vi "CreateNewProj.vi"() -> ()   [LabVIEW 2026]
panel:
  out "error out":errorcluster
  in  "error in (no error)":errorcluster
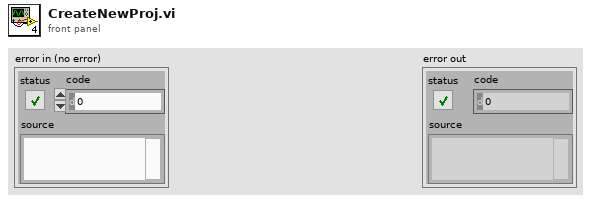
[diagram p1: front panel]
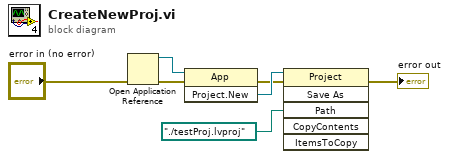
[diagram p0: block diagram]
diagram:
  n1 = Open Application Reference(8:"error in (no error)") -> (0:w3:errorcluster, 3:w7:refnum<vi>)  [unwired: 3 in]
  n2 = invoke class="App" method="Project.New"(reference=w7, error in=w3) -> (error out=w2:errorcluster, "Project:New"=w6:refnum<vi>)  [unwired: 1 in, 1 out]
  n3 = invoke class="Project" method="Save As"(reference=w6, error in=w2, "Path"=path "./testProj.lvproj") -> (error out=→"error out":errorcluster)  [unwired: 3 in, 5 out]
